vi "Prompt_FileExists.vi"(5 "Attempted File Path":path=path "C:/Labview Test Data/2018-08-07/0/Temp Dependence/Sensors_DAQ_200C_8.tdms", 6 "Measurement number":i32=8, 7 "Meas. Description":string="200C", 8 "SubFolder":string="Temp Dependence", 9 "Project":u16(ring)) -> (0 "Overwrite":bool=TRUE, 1 "Meas. Description 2":string="200C", 2 "SubFolder 2":string="Temp Dependence", 3 "Project 2":enum16{"H2TC", "VAPOR1"}(ring), 4 "Measurement number 2":i32=8)   [LabVIEW 2018]
doc: "Displays a standard dialog box that prompts users to enter information, such as a user name and password.\n--------------------\n\nThis Express VI is configured as follows:\n\nMessage to Display to the User:\nThe inputs are: \nText Entry Box: Project\nText Entry Box: Measurement Description\nNumber: Measurement Number"
panel:
  out "String 2":string="Change information below to generate unique filename or overwrite" caption="String"
  out "error out":errorcluster
  in  "error in (no error)":errorcluster
  in  "Enable":bool=TRUE
  in  "Cancel":bool
  in  "OK2":bool
  in  "OK1":bool
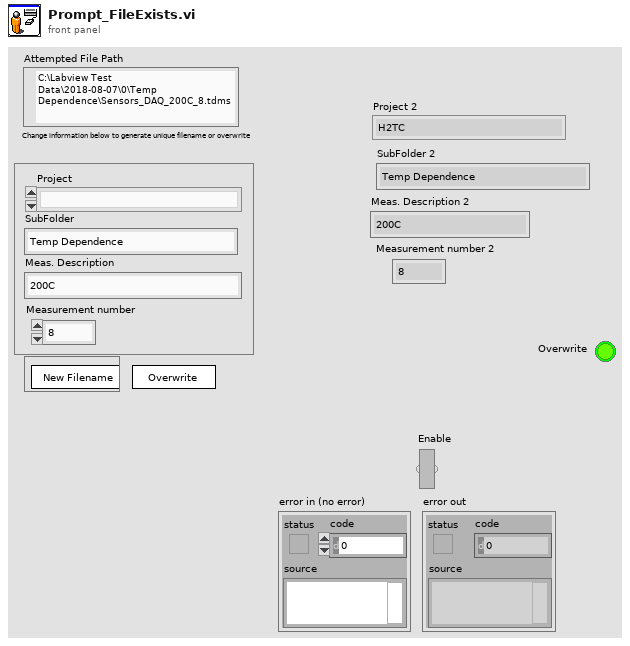
[diagram p1: front panel]
types:
  T1 = cluster{"Input Name":string, "Input Data Type":i32}[]
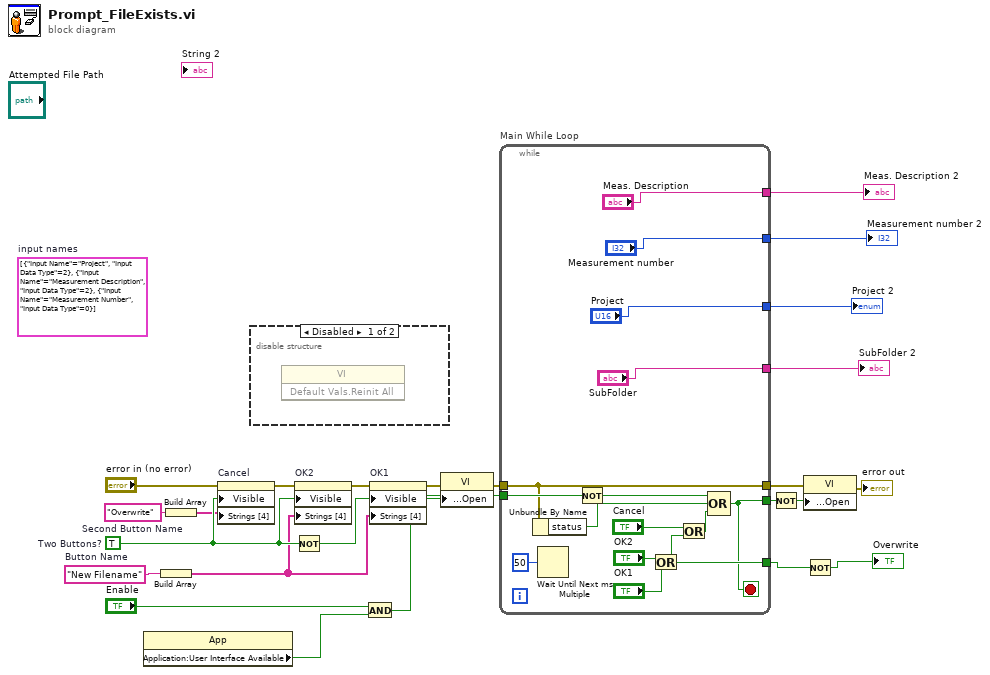
[diagram p0: block diagram]
diagram:
  (unwired) T1 [{"Input Name"="Project", "Input Data Type"=2}, {"Input Name"="Measurement Description", "Input Data Type"=2}, {"Input Name"="Measurement Number", "Input Data Type"=0}]  # input names
  w17 = "Overwrite"  # Second Button Name
  w15 = "New Filename"  # Button Name
  w24 = TRUE  # Two Buttons?
  n1 = property class="App"() -> ("Application:User Interface Available"=w7:bool)  [unwired: 2 in, 2 out]
  n2 = Build Array(w15) -> (w16:string[])
  n3 = Build Array(w17) -> (w18:string[])
  n4 = property on="Cancel" class="Bool"(error in="error in (no error)", "Visible"=w24, "Strings [4]"=w18) -> (error out=w22:errorcluster)  [unwired: 1 in, 1 out]
  n5 = disable-structure shown="Disabled" {
    frame Disabled {
      n6 = invoke class="VI" method="Default Vals.Reinit All"() -> ()  [unwired: 3 in, 3 out]
    }
    frame Enabled {
    }
  }
  n7 = Not(x=w24) -> (.not. x?=w23:bool)
  n8 = property on="OK2" class="Bool"(error in=w22, "Visible"=w24, "Strings [4]"=w16) -> (error out=w21:errorcluster)  [unwired: 1 in, 1 out]
  n9 = And(x="Enable", y=w7) -> (x .and. y?=w8:bool)
  n10 = property on="OK1" class="Bool"(error in=w21, "Visible"=w23, "Strings [4]"=w16) -> (error out=w14:errorcluster)  [unwired: 1 in, 1 out]
  n11 = property class="VI"(error in=w14, "Front Panel Window:Open"=w8) -> (error out=w13:errorcluster)  [unwired: 1 in, 1 out]
  n12 = while "Main While Loop" {
    tunnel: [w36] -> w6
    tunnel: w8 -> [w34]
    tunnel: [w32] -> w19
    tunnel: w13 -> [w31]
    tunnel: [w31] -> w11
    tunnel: ["Meas. Description"] -> w4
    tunnel: ["Measurement number"] -> w3
    tunnel: ["Project"] -> w2
    tunnel: ["SubFolder"] -> w1
    stop <- w32 stop-if-true
    n13 = Unbundle By Name(w31) -> ("status"=w29:bool)
    n14 = Wait Until Next ms Multiple(millisecond multiple=u32 50) -> ()  [unwired: 1 out]
    n15 = Not(x=w34) -> (.not. x?=w33:bool)
    n16 = Or(x="OK2", y="OK1") -> (x .or. y?=w36:bool)
    n17 = Or(x="Cancel", y=w36) -> (x .or. y?=w30:bool)
    n18 = Compound Arithmetic op=OR(w33, w29, w30) -> (w32:bool)
  }
  "Meas. Description 2" <- w4
  "Measurement number 2" <- w3
  "SubFolder 2" <- w1
  "Project 2" <- w2
  n19 = Not(x=w19) -> (.not. x?=w20:bool)
  n20 = property class="VI"(error in=w11, "Front Panel Window:Open"=w20) -> (error out=→"error out":errorcluster)  [unwired: 1 in, 1 out]
  n21 = Not(x=w6) -> (.not. x?=→"Overwrite":bool)
